vi "absolute_speed.vi"(1 "Wind Vector":cluster{"Wind R":dbl, "Wind Theta":dbl}, 2 "Boat Angle":dbl) -> (0 "Velocity":dbl)   [LabVIEW 2011]
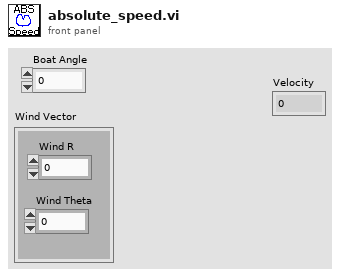
[diagram p1: front panel]
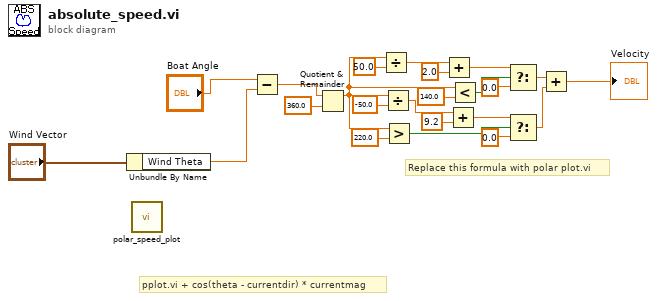
[diagram p0: block diagram]
diagram:
  # "Replace this formula with polar plot.vi"
  # "pplot.vi + cos(theta - currentdir) * currentmag"
  n1 = Unbundle By Name("Wind Vector") -> ("Wind Theta"=w19:dbl)
  n2 = call "polar_speed_plot.vi"() -> ()  [unwired: 2 in, 1 out]
  n3 = Subtract(x="Boat Angle", y=w19) -> (x-y=w22:dbl)
  n4 = Quotient & Remainder(x=w22, y=360.0) -> (x-y*floor(x/y)=w2:dbl)  [unwired: 1 out]
  n5 = Divide(x=w2, y=50.0) -> (x/y=w10:dbl)
  n6 = Divide(x=w2, y=-50.0) -> (x/y=w5:dbl)
  n7 = Greater?(x=w2, y=220.0) -> (0:w13:bool)
  n8 = Add(x=w10, y=2.0) -> (x+y=w11:dbl)
  n9 = Add(x=w5, y=9.2) -> (x+y=w3:dbl)
  n10 = Less?(x=w2, y=140.0) -> (x < y?=w17:bool)
  n11 = Select(t=w11, s=w17, f=0.0) -> (s? t:f=w8:dbl)
  n12 = Select(t=w3, s=w13, f=0.0) -> (s? t:f=w7:dbl)
  n13 = Add(x=w8, y=w7) -> (x+y=→"Velocity":dbl)
